vi "sendEmail.vi"(8 "error in (no error)":errorcluster, 9 "Recipient's Email Address Address":string="frouman@gmail.com", 10 "Queue Length":dbl, 11 "Acquisition in":refnum<class "Acquisition.lvclass">) -> (0 "error out":errorcluster, 3 "Acquisition out":refnum<class "Acquisition.lvclass">)   [LabVIEW 2014, in "Acquisition.lvclass"]
uses:
  Acquisition.lvclass
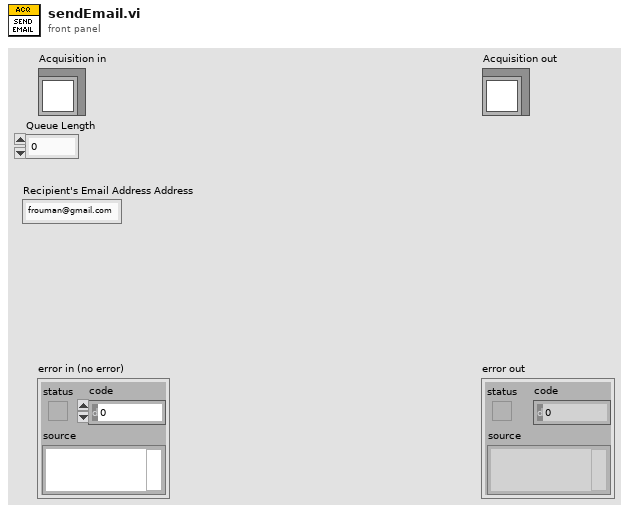
[diagram p1: front panel]
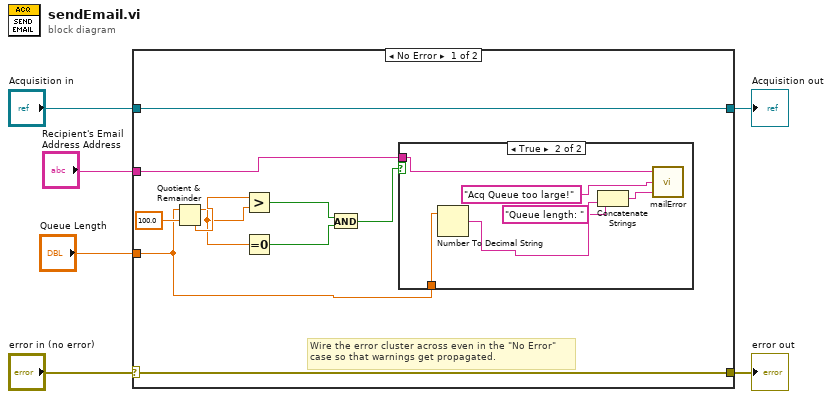
[diagram p0: block diagram]
diagram:
  n1 = case shown="No Error" "error in (no error)" {
    selector: "error in (no error)" -> [w15 w24]
    tunnel: [w15 w24] -> w5
    tunnel: [w16 w23] -> w3
    tunnel: "Acquisition in" -> [w16 w23]
    tunnel: "Queue Length" -> [w8 _]
    tunnel: "Recipient's Email Address Address" -> [w7 _]
    frame No Error {
      # "Wire the error cluster across even in the \"No Error\"\ncase so that warnings get propagated."
      n2 = Quotient & Remainder(x=w8, y=100.0) -> (x-y*floor(x/y)=w9:dbl, floor(x/y)=w10:dbl)
      n3 = Greater?(x=w10, y=w9) -> (0:w11:bool)
      n4 = Equal To 0?(x=w9) -> (x = 0?=w12:bool)
      n5 = And(x=w11, y=w12) -> (x .and. y?=w14:bool)
      n6 = case shown="True" w14 {
        tunnel: w8 -> [_ w22]
        tunnel: w7 -> [_ w17]
        frame False {
        }
        frame True {
          n7 = Number To Decimal String(number=w22) -> (decimal integer string=w21:string)  [unwired: 1 in]
          n8 = Concatenate Strings("Queue length: " ("string"), w21) -> (w19:string)
          n9 = call "mailError.vi"("Body"=w19, "Subject"="Acq Queue too large!", "Recipient's Email Address Address"=w17) -> ()  [unwired: 1 in]
        }
      }
    }
    frame Error {
    }
  }
  "error out" <- w5
  "Acquisition out" <- w3
